vi "SetzFarbe.vi"(10 "Farbfeld":u32(colorbox)=6618880, 11 "Array":refnum<vi>[](array[refnum])) -> (3 "Array 2":refnum<vi>[](array[refnum]))   [LabVIEW 2014]
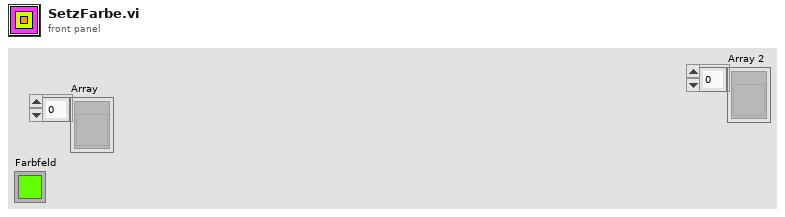
[diagram p1: front panel]
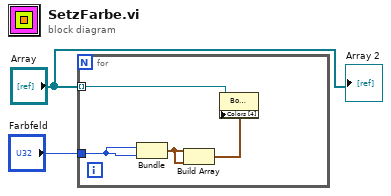
[diagram p0: block diagram]
diagram:
  n1 = for {
    tunnel: "Array" -> [w4] mode=indexing
    tunnel: "Farbfeld" -> [w3]
    n2 = Bundle("Farbfeld"=w3, "Farbfeld"=w3) -> (w6:cluster{"Farbfeld":u32, "Farbfeld":u32})  [unwired: 1 in]
    n3 = Build Array(w6, w6) -> (w5:cluster{"Farbfeld":u32, "Farbfeld":u32}[])
    n4 = property class="Bool. (strikt)"(reference=w4, "Colors [4]"=w5) -> ()  [unwired: 1 in, 2 out]
  }
  "Array 2" <- "Array"
